vi "BotStatus.vi"() -> ()   [LabVIEW 2012]
panel:
  in  "Cannon LS":T1
  in  "Frisbee in Stack Counter":i32
  in  "Cannon Min Angle CONST (deg)":dbl
  in  "Disable Stack":bool
  in  "Target Info":T2
  in  "Empty Stack":bool
  in  "Distance [m]":dbl
  in  "Climbing":bool
  in  "Cannon Position(deg)":dbl
  in  "Frisbee States":T3
  in  "Stow":bool
  # "Cannon"
  # "From end of cannon to center of target"
  # "InCannon"
  # "InFlipper"
  # "FlipperAtPlace"
  # "Middle"
  # "Bottom"
  # "UPDATES VALUES IN Periodic Tasks.vi"
  # "Feeder Angle"
  # "Flipper Angle"
  # "Cannon Angle"
  # "90"
  # "90"
  # "90"
  # "131"
  # "170"
  # "170"
  # "0"
  # "48.6 => 49"
  # "0"
  # "-min angle"
  # "0"
  # "\"Cannon Position(deg)\""
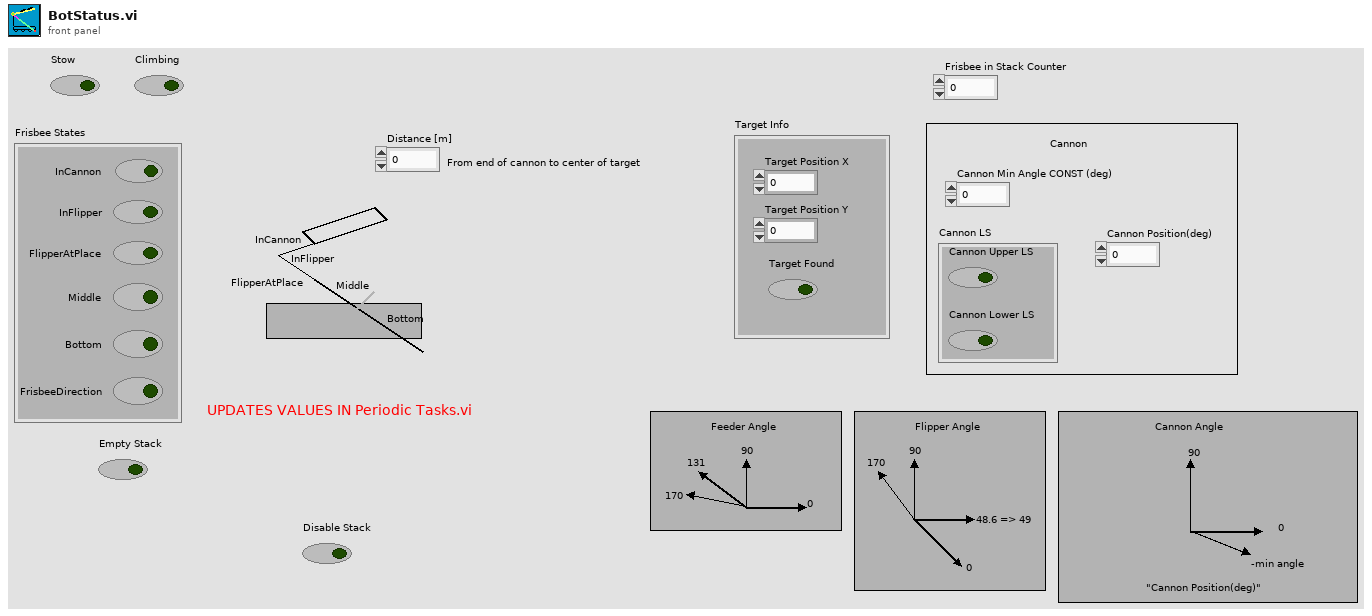
[diagram p1: front panel]
types:
  T1 = cluster{"Cannon Upper LS":bool, "Cannon Lower LS":bool}
  T2 = cluster{"Target Position X":dbl, "Target Position Y":dbl, "Target Found":bool}
  T3 = cluster{"Middle":bool, "InCannon":bool, "InFlipper":bool, "FlipperAtPlace":bool, "Bottom":bool, "FrisbeeDirection":bool}
diagram:
